vi "SwerveMath.vi"(0 "X-Axis":dbl, 2 "Y-Axis":dbl, 4 "Turn":dbl) -> (20 "FrontLeftAngle":dbl, 21 "FrontRightAngle":dbl, 22 "RearLeftAngle":dbl, 23 "RearRightAngle":dbl, 24 "FrontLeftDrive":dbl, 25 "FrontRightDrive":dbl, 26 "RearLeftDrive":dbl, 27 "RearRightDrive":dbl)   [LabVIEW 2018]
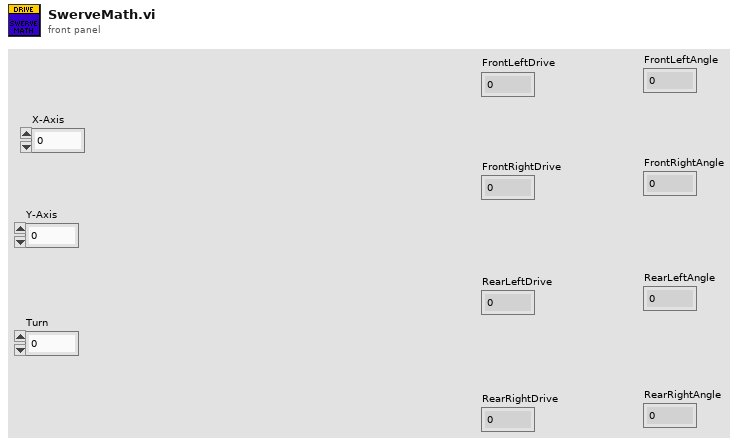
[diagram p1: front panel]
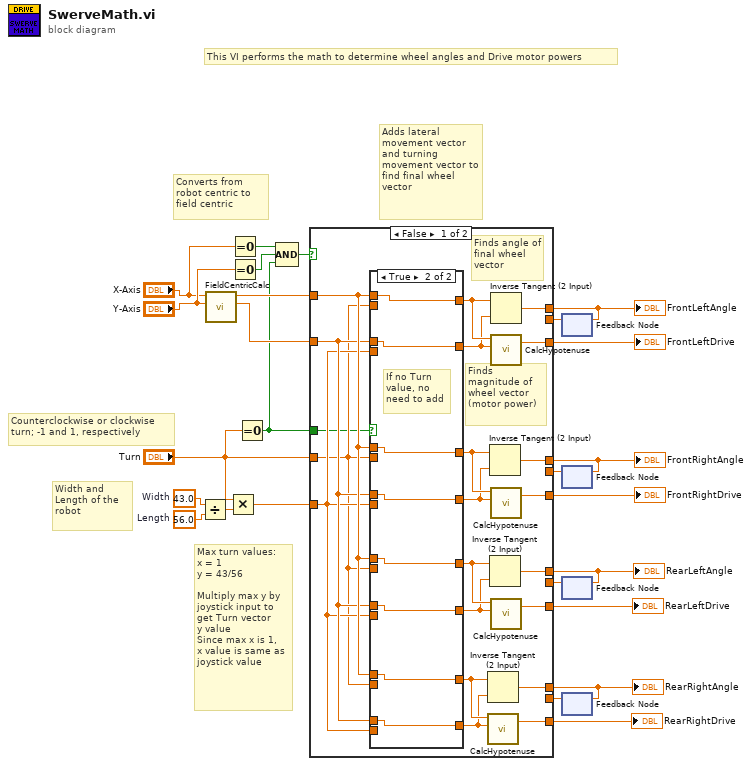
[diagram p0: block diagram]
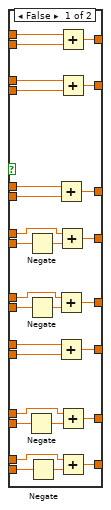
[diagram p2: hidden frame]
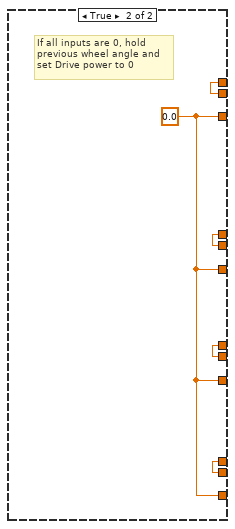
[diagram p3: hidden frame]
diagram:
  w24 = 56.0  # Length
  w25 = 43.0  # Width
  # "This VI performs the math to determine wheel angles and Drive motor powers"
  # "Adds lateral movement vector and turning movement vector to find final wheel vector"
  # "Width and Length of the robot"
  # "Converts from robot centric to field centric"
  # "Counterclockwise or clockwise turn; -1 and 1, respectively"
  # "Max turn values:\nx = 1\ny = 43/56\n\nMultiply max y by\njoystick input to\nget Turn vector\ny value\nSince max x is 1,\nx value is same as\njoystick value"
  n1 = Divide(x=w25, y=w24) -> (x/y=w23:dbl)
  n2 = call "FieldCentricCalc.vi"("y_in"="Y-Axis", "x_in"="X-Axis") -> ("y_out"=w17:dbl, "x_out"=w18:dbl)  [unwired: 8 in]
  n3 = Multiply(x="Turn", y=w23) -> (x*y=w16:dbl)
  n4 = Equal To 0?(x="X-Axis") -> (x = 0?=w10:bool)
  n5 = Equal To 0?(x="Y-Axis") -> (x = 0?=w9:bool)
  n6 = Equal To 0?(x="Turn") -> (x = 0?=w6:bool)
  n7 = Compound Arithmetic op=AND(w10, w9, w6) -> (w1:bool)
  n8 = feedback #1() -> (w5:dbl)  [unwired: 1 in]
  n9 = feedback #2() -> (w2:dbl)  [unwired: 1 in]
  n10 = feedback #3() -> (w4:dbl)  [unwired: 1 in]
  n11 = feedback #4() -> (w3:dbl)  [unwired: 1 in]
  n12 = case shown="False" w1 {
    tunnel: [w46 w83] -> w22
    tunnel: [w45 w83] -> w21
    tunnel: [w44 w83] -> w20
    tunnel: [w43 w83] -> w19
    tunnel: w18 -> [w42 _]
    tunnel: w17 -> [w33 _]
    tunnel: w16 -> [w32 _]
    tunnel: "Turn" -> [w31 _]
    tunnel: w6 -> [w30 _]
    tunnel: [w29 w85] -> w11
    tunnel: [w28 w86] -> w12
    tunnel: [w27 w84] -> w13
    tunnel: [w26 w87] -> w14
    tunnel: w5 -> [_ w87]
    tunnel: w4 -> [_ w86]
    tunnel: w3 -> [_ w85]
    tunnel: w2 -> [_ w84]
    frame False {
      # "Finds magnitude of wheel vector (motor power)"
      # "Finds angle of final wheel vector"
      n13 = case shown="True" w30 {
        tunnel: w42 -> [w70 w82]
        tunnel: w31 -> [w69 _]
        tunnel: w33 -> [w68 w81]
        tunnel: w32 -> [w67 _]
        tunnel: w42 -> [w66 w80]
        tunnel: w31 -> [w65 _]
        tunnel: w33 -> [w64 w79]
        tunnel: w32 -> [w63 _]
        tunnel: w31 -> [w62 _]
        tunnel: w42 -> [w61 w78]
        tunnel: w33 -> [w60 w77]
        tunnel: w32 -> [w59 _]
        tunnel: w42 -> [w58 w76]
        tunnel: w31 -> [w57 _]
        tunnel: w33 -> [w56 w75]
        tunnel: w32 -> [w55 _]
        tunnel: [w54 w82] -> w41
        tunnel: [w53 w81] -> w40
        tunnel: [w52 w80] -> w39
        tunnel: [w51 w79] -> w38
        tunnel: [w50 w78] -> w37
        tunnel: [w49 w77] -> w36
        tunnel: [w48 w76] -> w35
        tunnel: [w47 w75] -> w34
        frame False {
          n14 = Negate(x=w57) -> (-x=w71:dbl)
          n15 = Negate(x=w63) -> (-x=w74:dbl)
          n16 = Negate(x=w62) -> (-x=w73:dbl)
          n17 = Negate(x=w55) -> (-x=w72:dbl)
          n18 = Add(x=w66, y=w65) -> (x+y=w52:dbl)
          n19 = Add(x=w61, y=w73) -> (x+y=w50:dbl)
          n20 = Add(x=w60, y=w59) -> (x+y=w49:dbl)
          n21 = Add(x=w64, y=w74) -> (x+y=w51:dbl)
          n22 = Add(x=w70, y=w69) -> (x+y=w54:dbl)
          n23 = Add(x=w68, y=w67) -> (x+y=w53:dbl)
          n24 = Add(x=w58, y=w71) -> (x+y=w48:dbl)
          n25 = Add(x=w56, y=w72) -> (x+y=w47:dbl)
        }
        frame True {
          # "If no Turn value, no need to add"
        }
      }
      n26 = Inverse Tangent (2 Input)(1:w34, 2:w35) -> (0:w29:dbl)
      n27 = call "CalcHypotenuse.vi"("b"=w34, "a"=w35) -> ("hypotenuse"=w46:dbl)  [unwired: 3 in]
      n28 = Inverse Tangent (2 Input)(1:w38, 2:w39) -> (0:w27:dbl)
      n29 = Inverse Tangent (2 Input)(1:w36, 2:w37) -> (0:w28:dbl)
      n30 = Inverse Tangent (2 Input)(1:w40, 2:w41) -> (0:w26:dbl)
      n31 = call "CalcHypotenuse.vi"("b"=w40, "a"=w41) -> ("hypotenuse"=w43:dbl)  [unwired: 3 in]
      n32 = call "CalcHypotenuse.vi"("b"=w38, "a"=w39) -> ("hypotenuse"=w44:dbl)  [unwired: 3 in]
      n33 = call "CalcHypotenuse.vi"("b"=w36, "a"=w37) -> ("hypotenuse"=w45:dbl)  [unwired: 3 in]
    }
    frame True {
      w83 = 0.0 ("hypotenuse")
      # "If all inputs are 0, hold previous wheel angle and set Drive power to 0"
    }
  }
  "FrontLeftAngle" <- w14
  "FrontRightAngle" <- w13
  "RearLeftAngle" <- w12
  "RearRightAngle" <- w11
  "FrontLeftDrive" <- w19
  "FrontRightDrive" <- w20
  "RearLeftDrive" <- w21
  "RearRightDrive" <- w22
  n34 = feedback-in #1(w14) -> ()
  n35 = feedback-in #2(w13) -> ()
  n36 = feedback-in #3(w12) -> ()
  n37 = feedback-in #4(w11) -> ()
